vi "Write Key (String).vi"(6 "Write Raw String? (F)":bool, 7 "Section Name":string, 8 "error in (no error)":errorcluster, 9 "Value":string, 10 "Key Name":string, 11 "Config in":T1) -> (0 "error out":errorcluster, 2 "Key Replaced?":bool, 3 "Config out":T1)   [LabVIEW 2022 SP3, in "LabVIEW-Config.lvlib"]
uses:
  LabVIEW-Config.lvlib
  Config.ctl
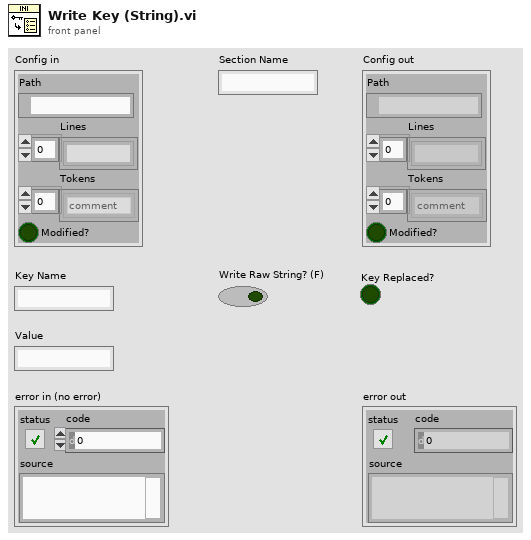
[diagram p1: front panel]
types:
  T1 = typedef "LabVIEW-Config.lvlib/Config.ctl" = cluster{"Path":path, "Lines":string[], "Tokens":enum8{"comment", "section", "key"}[], "Modified?":bool}
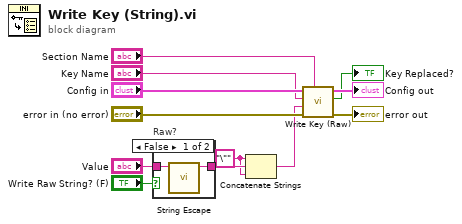
[diagram p0: block diagram]
diagram:
  w1 = "\"" ("string")
  n1 = case "Raw?" shown="False" "Write Raw String? (F)" {
    tunnel: "Value" -> [w14 w15]
    tunnel: [w13 w15] -> w3
    frame False {
      n2 = call "String Escape.vi"("Unescaped String"=w14) -> ("Escaped String"=w13:string)  [unwired: 10 in]
    }
    frame True {
    }
  }
  n3 = Concatenate Strings(w1, w3, w1) -> (w2:string)
  n4 = call "Write Key (Raw).vi"("Section Name"="Section Name", "error in (no error)"="error in (no error)", "Content"=w2, "Key Name"="Key Name", "Config in"="Config in") -> ("error out"=→"error out":errorcluster, "Key Replaced?"=→"Key Replaced?":bool, "Config out"=→"Config out":T1)  [unwired: 4 in]
